vi "2 dr_dt.vi"(1 "Apparent Wind\nSpeed":T1, 2 "Apparent Wind\nDirection (º)":T2, 3 "Boat Angle":dbl) -> (0 "dr/dt":dbl)   [LabVIEW 2011]
doc: "Given a wind vector and boat angle, returns the speed that the boat will approach the goal (assuming that the goal is at 0 degrees). This simply uses the estimated speed based on wind, and the cosine of the boat angle."
uses:
  2 Typedefs/apparent wind direction.ctl
  2 Typedefs/apparent wind speed.ctl
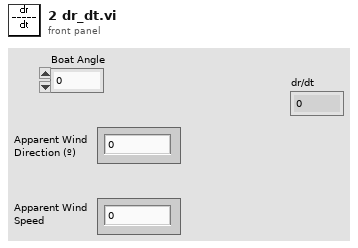
[diagram p1: front panel]
types:
  T1 = typedef "apparent wind speed.ctl" = dbl
  T2 = typedef "apparent wind direction.ctl" = dbl
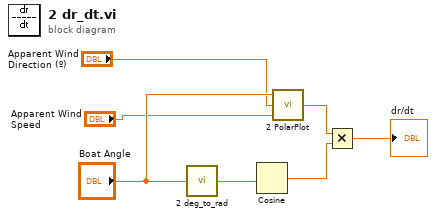
[diagram p0: block diagram]
diagram:
  n1 = call "2 deg_to_rad.vi"("Degrees"="Boat Angle") -> ("Radians"=w7:dbl)
  n2 = Cosine(x=w7) -> (cos(x)=w4:dbl)
  n3 = call "2 PolarPlot.vi"("Apparent Wind\nSpeed"="Apparent Wind\nSpeed", "Apparent Wind\nDirection (º)"="Apparent Wind\nDirection (º)", "Boat Angle"="Boat Angle") -> ("Velocity"=w6:dbl)
  n4 = Multiply(x=w6, y=w4) -> (x*y=→"dr/dt":dbl)
